vi "Lab4_1.vi"(4 "n":dbl) -> (0 "Nmin":dbl, 1 "Результат":dbl, 2 "Nmax":dbl)   [LabVIEW 2011]
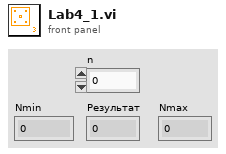
[diagram p1: front panel]
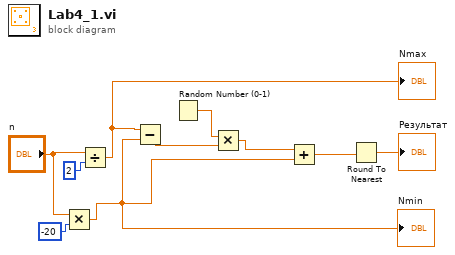
[diagram p0: block diagram]
diagram:
  n1 = Multiply(x="n", y=-20) -> (x*y=w2:dbl)
  "Nmin" <- w2
  n2 = Divide(x="n", y=2) -> (x/y=w1:dbl)
  "Nmax" <- w1
  n3 = Subtract(x=w1, y=w2) -> (x-y=w3:dbl)
  n4 = Random Number (0-1)() -> (number: 0 to 1=w4:dbl)
  n5 = Multiply(x=w4, y=w3) -> (x*y=w5:dbl)
  n6 = Add(x=w5, y=w2) -> (x+y=w6:dbl)
  n7 = Round To Nearest(number=w6) -> (nearest integer value=→"Результат":dbl)
